vi "Update Hardware Configuration File Error.vi"(8 "error in":errorcluster, 11 "Configuration files Ref":T1 format="%.0x") -> (0 "error out":errorcluster, 3 "Configuration files Ref out":T1 format="%.0x")   [LabVIEW 2020, in "Ballard ARINC 429 System Explorer.lvlib" / "Implementation.lvlib"]
uses:
  Implementation.lvlib
  Scripting/Ballard ARINC 429 Scripting.lvlib
  <vilib>/NI VeriStand/Custom Device API/Custom Device Item Ref.ctl
  <vilib>/NI VeriStand/Custom Device API/Custom Device API.lvlib
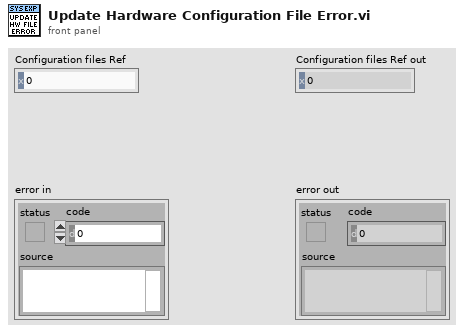
[diagram p1: front panel]
types:
  T1 = typedef "Custom Device API.lvlib/Custom Device Item Ref.ctl" = u64
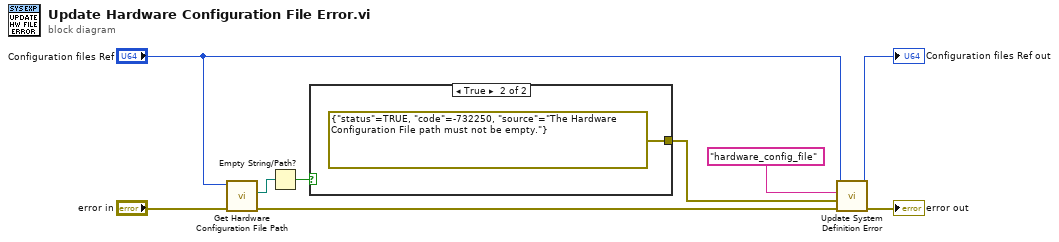
[diagram p0: block diagram]
diagram:
  n1 = call "Get Hardware Configuration File Path.vi"("error in"="error in", "Configuration files Ref"="Configuration files Ref") -> ("error out"=w5:errorcluster, "Path"=w2:path)  [unwired: 7 in, 1 out]
  n2 = Empty String/Path?(string/path=w2) -> (empty?=w6:bool)
  n3 = case shown="True" w6 {
    tunnel: [_ errorcluster {"status"=TRUE, "code"=-732250, "source"="The Hardware Configuration File path must not be empty."} ("New Error")] -> w4
    frame False {
    }
    frame True {
    }
  }
  n4 = call "Update System Definition Error.vi"("error to report"=w5, "error in"=w4, "error key"="hardware_config_file", "Configuration files Ref"="Configuration files Ref") -> ("error out"=→"error out":errorcluster, "Configuration files Ref out"=→"Configuration files Ref out":T1)  [unwired: 6 in]
